vi "SendToDb.vi"(0 "reference in":refnum<class "NeedleValve.lvclass">, 11 "error in (no error)":errorcluster) -> (4 "reference out":refnum<class "NeedleValve.lvclass">, 15 "error out":errorcluster)   [LabVIEW 2019, in "NeedleValve.lvclass"]
uses:
  NeedleValve.lvclass
  D:/GIT H4000/H4000/src/Proccess_class/Proccess.lvclass
  NeedleValve.lvclass/NeedleValve.ctl
  Proccess_class/Proccess.lvclass/Proccess.ctl
  Logger_class/EventData.ctl
  TypeDef/AlarmType.ctl
  ddaf1088-39ed-46bc-a000-2f82a45c55df.vi
  Logger_class/Logger.lvclass
  Proccess_class/Proccess.lvclass
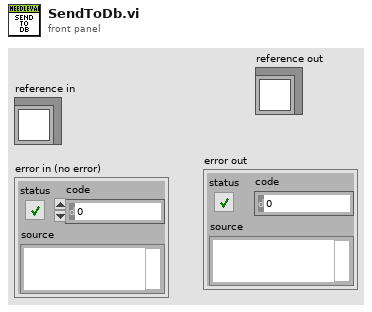
[diagram p1: front panel]
types:
  T1 = typedef "Needle Valve Data.ctl" = cluster{"Engine State":T2, "StateValveModbus":T3, "Alarms":T4, "RAW":i32, "Angele":dbl, "Step":i32, "Encoder":i32, "Kinematic":T5, "Limits":T6, "EncoderMax":i32, "Counter Max Dont Update":i32, "EncoderMin":i32, "Counter Min Dont Update":i32, "Prepere Counter":i32, "STEP INIT":i32, "offset - Angel":dbl}
  T2 = typedef "MB_ENGINE.lvclass/Engine State.ctl" = u16
  T3 = typedef "Needle Valve State.ctl" = enum16{"STOPED", "CLOSED", "OPENED", "OPENING", "CLOSING", "FULL_CLOSE", "PREP_OPEN"}
  T4 = typedef "MB_ENGINE.lvclass/Engine Alarms.ctl" = cluster{"OL":bool, "TF":bool, "STL":bool, "OCP":bool, "CPUV":bool, "UVLO":bool, "SPI_ERROR":bool, "Fault":bool, "OL 2":bool, "TF 2":bool, "STL 2":bool, "OCP 2":bool, "CPUV 2":bool, "UVLO 2":bool, "reserved":bool, "InitDone":bool}
  T5 = typedef "MB_ENGINE.lvclass/Settings.ctl" = cluster{"ACC Steps Per Sec^2":u16, "DEC Steps Per Sec^2":u16, "Min Velosity Step Per Sec":u16, "Max Velosity Step Per Sec":u16, "MicroStep":u16}
  T6 = typedef "MB_ENGINE.lvclass/Limits Status.ctl" = cluster{"Fault 2 Switch":bool, "Fault 1 Switch":bool, "Center(Home)":bool, "Lower Limit":bool, "Upper Limit":bool}
  T7 = typedef "EventData.ctl" = cluster{"obj_tag":string, "event_tag":string, "Description":string, "ALARM TYPE":T8, "Value DBL":dbl, "Value INT":i32, "Value STR":string, "Time Stamp":timestamp}
  T8 = typedef "AlarmType.ctl" = enum16{"Normal", "Warning", "Alarm"}
  T9 = typedef "Proccess.lvclass/TAGs.ctl" = cluster{"TAG":string, "PTAG":string, "DESC":string}
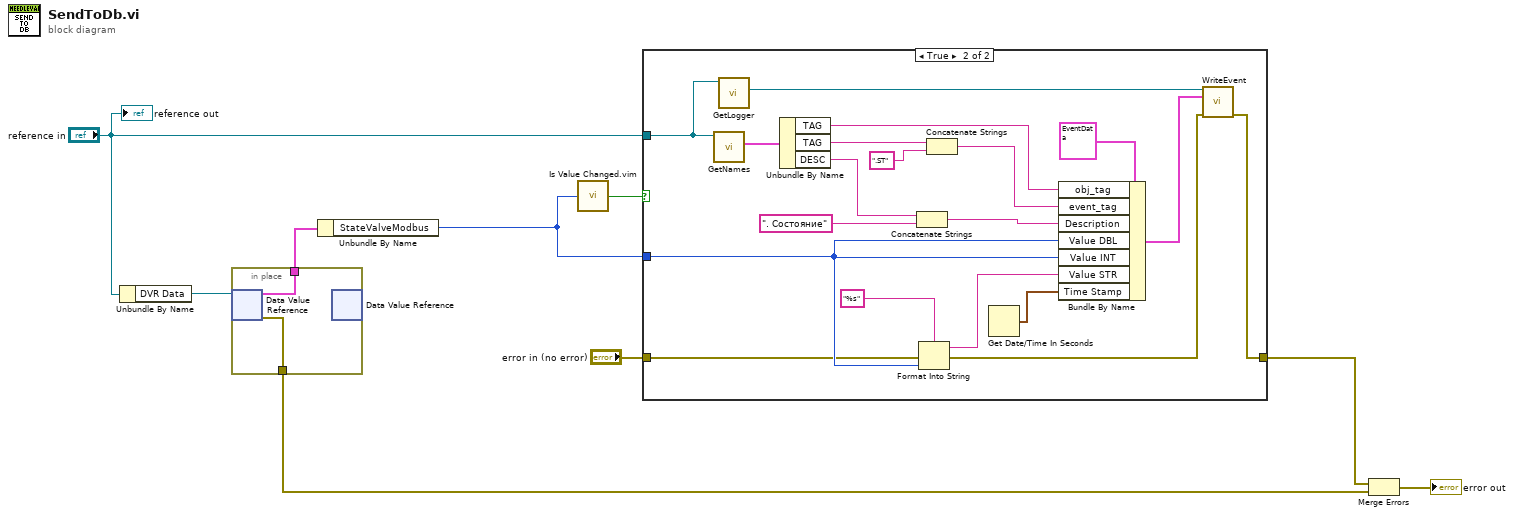
[diagram p0: block diagram]
diagram:
  n1 = Unbundle By Name("reference in") -> ("DVR Data"=w5:refnum<data-value>)
  n2 = in-place {
    in-place-border: [w11] -> w1
    in-place-border: [w10] -> w3
    n3 = in-place-dvr #1(w5) -> (w10:T1, w11:errorcluster)
    n4 = in-place-dvr #1() -> ()  [unwired: 1 in, 2 out]
  }
  n5 = Unbundle By Name(w3) -> ("StateValveModbus"=w7:T3)
  n6 = call "Is Value Changed.vim"("value"=w7) -> ("changed or first call?"=w6:bool)
  n7 = case shown="True" w6 {
    tunnel: [w12 w31] -> w9
    tunnel: "reference in" -> [_ w25]
    tunnel: w7 -> [_ w18]
    tunnel: "error in (no error)" -> [w12 w13]
    frame False {
    }
    frame True {
      n8 = call "GetNames.vi"("Proccess in"=w25) -> ("Tags"=w24:T9)  [unwired: 10 in]
      n9 = call "GetLogger.vi"("Proccess in"=w25) -> ("Logger"=w26:refnum<class "Logger.lvclass">)  [unwired: 10 in]
      n10 = Unbundle By Name(w24) -> ("TAG"=w23:string, "TAG"=w22:string, "DESC"=w21:string)
      n11 = Concatenate Strings(w21, ". Состояние" ("string")) -> (w15:string)
      n12 = Format Into String(format string="%s", error in=w13, w18) -> (resulting string=w17:string, error out=w16:errorcluster)  [unwired: 1 in]
      n13 = Concatenate Strings(w22, ".ST" ("string")) -> (w28:string)
      n14 = Get Date/Time In Seconds() -> (seconds since 1Jan1904=w20:timestamp)
      n15 = Bundle By Name(cluster=T7 {"obj_tag"="", "event_tag"="", "Description"="", "ALARM TYPE"=enum."Normal", "Value DBL"=0.0, "Value INT"=0, "Value STR"="", "Time Stamp"=timestamp(0 s since 1904-01-01)} ("Event"), "obj_tag"=w23, "event_tag"=w28, "Description"=w15, "Value DBL"=w18, "Value INT"=w18, "Value STR"=w17, "Time Stamp"=w20) -> (w30:T7)
      n16 = call "WriteEvent.vi"("reference in"=w26, "Event"=w30, "error in (no error)"=w16) -> ("error out"=w31:errorcluster)  [unwired: 11 in, 1 out]
    }
  }
  n17 = Merge Errors(w9, w1) -> (→"error out":errorcluster)
  "reference out" <- "reference in"
